vi "Calculate Record Beatable Counts.vi"(1 "Distances":string, 2 "Times":string) -> (0 "Record Beatable Counts":i32[](array[numeric]))   [LabVIEW 2020, in "AoC 2023.lvlib"]
uses:
  AoC 2023.lvlib
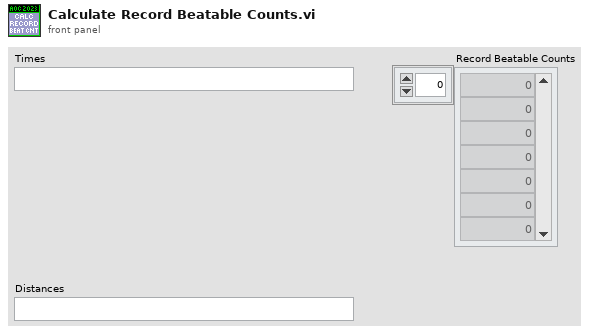
[diagram p1: front panel]
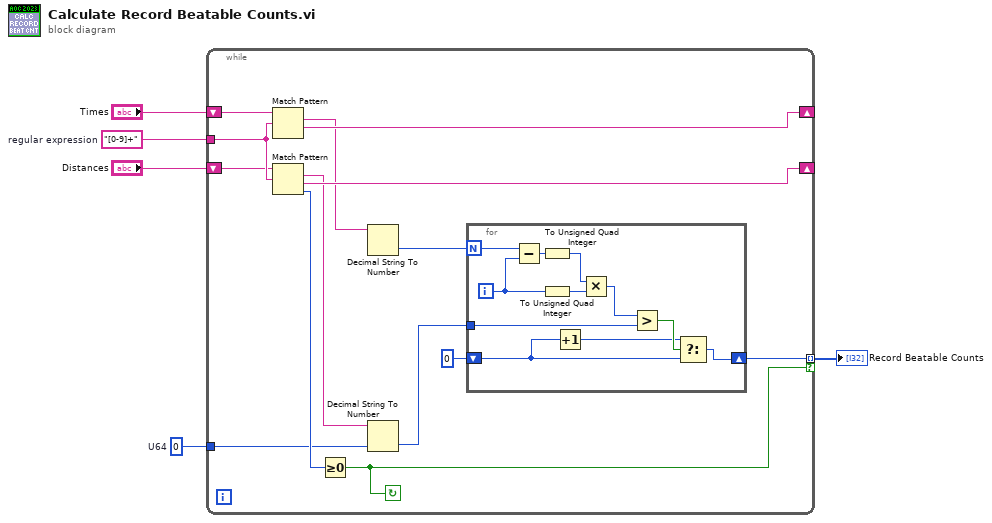
[diagram p0: block diagram]
diagram:
  w1 = u64 0  # U64
  w3 = "[0-9]+"  # regular expression
  n1 = while {
    tunnel: w3 -> [w17]
    shift-right: [w18] -> _
    shift-left: "Times" -> [w19]
    shift-right: [w15] -> _
    shift-left: "Distances" -> [w16]
    tunnel: [w8] -> w5 mode=indexing if=w6
    tunnel: w1 -> [w7]
    stop <- w6 continue-if-true
    n2 = Match Pattern(string=w19, regular expression=w17) -> (match substring=w13:string, after substring=w18:string)  [unwired: 1 in, 2 out]
    n3 = Match Pattern(string=w16, regular expression=w17) -> (match substring=w12:string, after substring=w15:string, offset past match=w14:i32)  [unwired: 1 in, 1 out]
    n4 = Greater Or Equal To 0?(x=w14) -> (x >= 0?=w6:bool)
    n5 = Decimal String To Number(string=w13) -> (number=w11:i32)  [unwired: 2 in, 1 out]
    n6 = Decimal String To Number(string=w12, default (0L)=w7) -> (number=w10:u64)  [unwired: 1 in, 1 out]
    n7 = for {
      N: w11 -> [w30]
      tunnel: w10 -> [w27]
      shift-right: [w24] -> w8
      shift-left: 0 -> [w23]
      i -> [w29]
      n8 = Subtract(x=w30, y=w29) -> (x-y=w28:i32)
      n9 = To Unsigned Quad Integer(1:w28) -> (0:w20:u64)
      n10 = To Unsigned Quad Integer(1:w29) -> (0:w21:u64)
      n11 = Increment(x=w23) -> (x+1=w22:i32)
      n12 = Multiply(x=w20, y=w21) -> (x*y=w26:u64)
      n13 = Greater?(x=w26, y=w27) -> (0:w25:bool)
      n14 = Select(t=w22, s=w25, f=w23) -> (s? t:f=w24:i32)
    }
  }
  "Record Beatable Counts" <- w5
